vi "Top Level Vi.vi"() -> ()   [LabVIEW 2015]
uses:
  Circle/Circle.lvclass
  Shape/Shape.lvclass
  Square/Square.lvclass
panel:
  out "Array":dbl[](array[numeric])
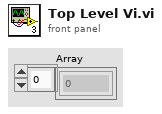
[diagram p1: front panel]
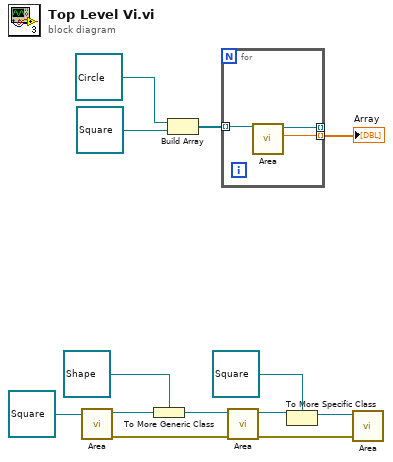
[diagram p0: block diagram]
diagram:
  n1 = call-dynamic "Area.vi"("Square in"=refnum<class "Square.lvclass"> refnum ("Square.lvclass")) -> ("error out"=w2:errorcluster, "Square out"=w5:refnum<class "Square.lvclass">)  [unwired: 8 in, 1 out]
  n2 = To More Generic Class(target class=refnum<class "Shape.lvclass"> refnum ("Circle.lvclass"), reference=w5) -> (generic class reference=w9:refnum<class "Shape.lvclass">)
  n3 = Build Array(refnum<class "Circle.lvclass"> refnum ("Circle.lvclass"), refnum<class "Square.lvclass"> refnum ("Square.lvclass")) -> (w13:refnum<class "Shape.lvclass">[])
  n4 = for {
    tunnel: w13 -> [w16] mode=indexing
    tunnel: [w15] -> _ mode=indexing
    tunnel: [w14] -> w12 mode=indexing
    n5 = call-dynamic "Area.vi"("Shape in"=w16) -> ("Numeric"=w14:dbl, "Shape out"=w15:refnum<class "Shape.lvclass">)  [unwired: 8 in, 1 out]
  }
  "Array" <- w12
  n6 = call-dynamic "Area.vi"("error in (no error)"=w2, "Shape in"=w9) -> ("error out"=w1:errorcluster, "Shape out"=w8:refnum<class "Shape.lvclass">)  [unwired: 7 in, 1 out]
  n7 = To More Specific Class(target class=refnum<class "Square.lvclass"> refnum ("Square.lvclass"), reference=w8) -> (specific class reference=w7:refnum<class "Square.lvclass">)  [unwired: 1 in, 1 out]
  n8 = call-dynamic "Area.vi"("error in"=w1, "Square in"=w7) -> ()  [unwired: 7 in, 3 out]
